vi "Write File+ [I16].vi"(6 "1D array":i16[](array[numeric]) caption="1D-Array", 7 "2D array":i16[][](array[numeric]) caption="2D-Array", 8 "error in (no error)":errorcluster caption="Fehler (Eingang, kein Fehler)", 9 "pos offset (bytes:0)":i32 caption="Pos.-Offset (Bytes:0)", 10 "pos mode (rel. to end:1)":enum16{"start", "end", "current"}(ring)=enum."end" caption="Pos.-Modus (relativ zum Ende:1)", 11 "refnum":refnum<file> caption="RefNum") -> (0 "error out":errorcluster caption="Fehler (Ausgang)", 1 "mark after write (bytes)":i32 caption="Dateimarke nach Schreibvorgang (Zeichen)", 3 "dup refnum":refnum<file> caption="RefNum (Kopie)")   [LabVIEW 2009]
doc: "Schreibt ein 2D- oder 1D-Array von vorzeichenbehafteten Word-Integerzahlen (I16) an der angegebenen Position in einer Byte-Stream-Datei; der voreingestellte Ort ist die aktuelle Markierung. Das VI überprüft eingehende und interne Fehler und schreibt nicht, wenn ein Eingangsfehler auftritt.\n\n'RefNum' ist die Referenz zur geöffneten Datei.\n\n'Pos.-Modus' legt fest, an welcher Stelle, relativ zu 'Pos.-Offset', zu schreiben begonnen wird:\n\n 0: am Anfang der Datei plus Pos.-Offest.\n\n 1: am Ende der Datei plus Pos.-Offest. Dies ist die Standardeinstellung.\n\n 2: an der aktuellen Markierung plus Pos.-Offset.\n\n'Pos.-Offset' legt in Byte fest, wie weit entfernt von 'Pos.-Modus' begonnen wird. Die Voreinstellung ist 0. Byte Einheiten sind flexibler als Integer (2 Byte) Einheiten, Wenn eine Datei zum Beispiel einen Kopf, geschrieben mit Datei Schreiben+ (String) enthält, gefolgt von Array mit Zahlen aus Datei Schreiben+ [I16].\n\n2D-Array enthält vorzeichenbehafteten Word-Integerzahlen, die das VI in die Datei schreibt, wenn das1D-Array nicht verbunden oder leer ist.\n\n1D Array enthält die vorzeichenbehafteten Word-Integerzahlen, die das VI in die Datei schreibt, wenn dieser Eingang nicht leer ist.\n\nFehlereingang ist ein Cluster mit 3 Elementen (Fehler?, Code, und Quelle) welches die Fehler des Speichervorganges anzeigt. Das VI kann nur dann normal ausgeführt werden, wenn kein Eingangsfehler vorliegt. Das VI kann nur dann normal ausgeführt werden, wenn kein Eingangsfehler vorliegt; sonst wird der vorher aufgetretene Fehler weitergeleitet. Fehler? ist TRUE, wenn ein Fehler aufgetreten ist; die Voreinstellung ist FALSE. Code ist der Fehlercode; die Voreinstellung ist 0. Quelle ist in den meisten Fällen der Name des VIs oder der Funktion in welcher der Fehler aufgetreten ist; die Voreinstellung ist ein leerer String. \n\nRefNum (Kopie) leitet die Referenznummer weiter.\n\nDateimarke nach Schreibvorgang siehe oben.\n\nFehlerausgang ist ein Cluster mit 3 Elementen (Fehler?, Code, und Quelle) welches den Fehlerstatus nach Ablauf des VIs beschreibt. Wenn kein Eingangsfehler auftrat, wird das VI normal ausgeführt und der Fehlerausgang enthält den Fehlerstatus dieses VIs; wenn ein Eingangsfehler auftrat wird diesen an den Fehlerausgang weitergegeben."
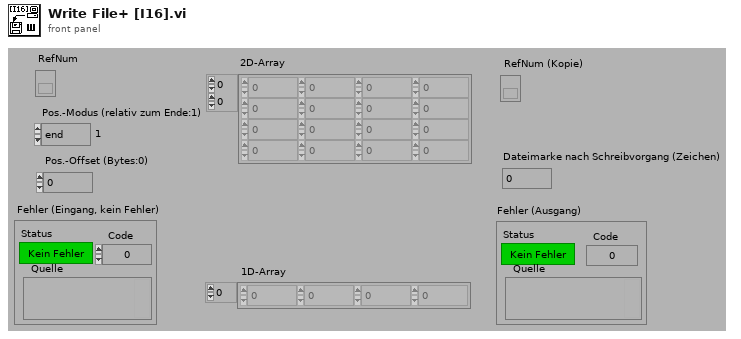
[diagram p1: front panel]
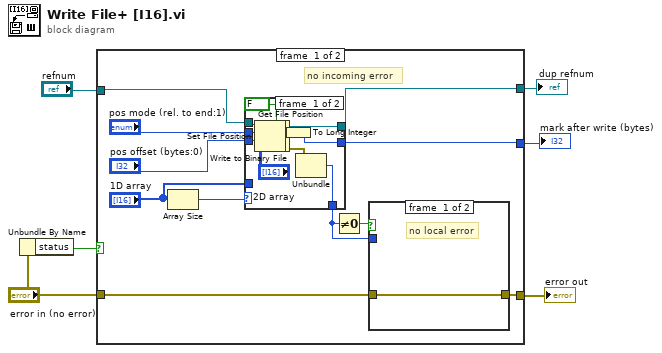
[diagram p0: block diagram]
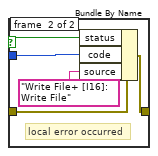
[diagram p2: hidden frame]
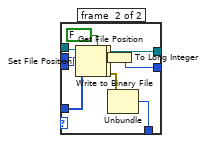
[diagram p3: hidden frame]
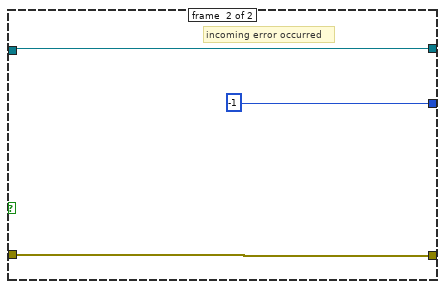
[diagram p4: hidden frame]
diagram:
  n1 = Unbundle By Name("error in (no error)") -> ("status"=w6:bool)
  n2 = case shown="False" w6 {
    tunnel: [w9 w53] -> w5
    tunnel: [w11 -1] -> w2
    tunnel: [w13 w52] -> w4
    tunnel: "refnum" -> [w14 w52]
    tunnel: "error in (no error)" -> [w10 w53]
    frame #0 {
      # "no incoming error"
      n3 = Array Size(array="1D array") -> (size(s)=w17:i32)
      n4 = case shown="..0" w17 {
        tunnel: "1D array" -> [_ w51]
        tunnel: "pos mode (rel. to end:1)" -> [w30 w44]
        tunnel: "pos offset (bytes:0)" -> [w36 w47]
        tunnel: w14 -> [w35 w48]
        tunnel: [w34 w50] -> w13
        tunnel: [w33 w49] -> w11
        tunnel: [w31 w46] -> w8
        frame #0 {
          n5 = Set File Position(offset (in bytes) (0)=w36, refnum=w35, from (0:start)=w30) -> (refnum out=w29:refnum<file>, error out=w28:errorcluster)  [unwired: 1 in]
          n6 = Write to Binary File(file (use dialog)=w29, data="2D array", error in=w28, 5:FALSE ("prepend array or string size? (T)")) -> (refnum out=w27:refnum<file>, error out=w26:errorcluster)  [unwired: 2 in, 1 out]
          n7 = Get File Position(4:w26, 7:w27) -> (0:w32:errorcluster, 2:w25:i64, 3:w34:refnum<file>)
          n8 = To Long Integer(number=w25) -> (32bit integer=w33:i32)
          n9 = Unbundle(w32) -> ("code"=w31:i32)  [unwired: 2 out]
        }
        frame #1 {
          n10 = Set File Position(offset (in bytes) (0)=w47, refnum=w48, from (0:start)=w44) -> (refnum out=w43:refnum<file>, error out=w42:errorcluster)  [unwired: 1 in]
          n11 = Write to Binary File(file (use dialog)=w43, data=w51, error in=w42, 5:FALSE ("prepend array or string size? (T)")) -> (refnum out=w41:refnum<file>, error out=w40:errorcluster)  [unwired: 2 in, 1 out]
          n12 = Get File Position(4:w40, 7:w41) -> (0:w45:errorcluster, 2:w39:i64, 3:w50:refnum<file>)
          n13 = To Long Integer(number=w39) -> (32bit integer=w49:i32)
          n14 = Unbundle(w45) -> ("code"=w46:i32)  [unwired: 2 out]
        }
      }
      n15 = Not Equal To 0?(x=w8) -> (x != 0?=w7:bool)
      n16 = case shown="True" w7 {
        selector: w7 -> [_ w19]
        tunnel: w8 -> [_ w22]
        tunnel: [w18 w23] -> w9
        tunnel: w10 -> [w18 w20]
        frame #0 {
          # "no local error"
        }
        frame #1 {
          # "local error occurred"
          n17 = Bundle By Name(cluster=w20, "status"=w19, "code"=w22, "source"="Write File+ [I16]: Write File") -> (w23:errorcluster)
        }
      }
    }
    frame #1 {
      # "incoming error occurred"
    }
  }
  "error out" <- w5
  "mark after write (bytes)" <- w2
  "dup refnum" <- w4
